vi "Project Parser.vi"(8 "error in (no error)":errorcluster, 10 "Initial Ident":i32, 11 "file path (use dialog)":path=path "C:/Users/fflores/Documents/LabVIEW Data/cRIO WFM/RT/Shared Variables/Local Variables.lvlib") -> (0 "error out":errorcluster, 2 "Item out":T1(array[cluster]))   [LabVIEW 2020, in "LV Project Items Parser.lvlib"]
doc: "This VI applies recursiveness to parse the elements of a project using its XML and return them ready to populate a tree control."
uses:
  LV Project Items Parser.lvlib
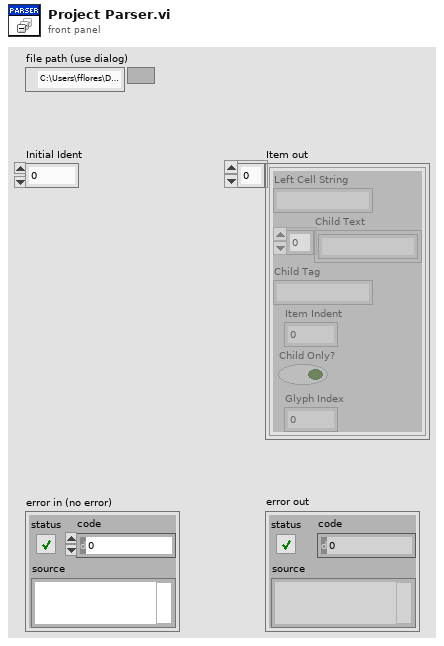
[diagram p1: front panel]
types:
  T1 = cluster{"Left Cell String":string, "Child Text":string[], "Child Tag":string, "Item Indent":i32, "Child Only?":bool, "Glyph Index":i32}[]
  T2 = cluster{"Left Cell String":string, "Child Text":string[], "Child Tag":string, "Item Indent":i32, "Child Only?":bool, "Glyph Index":i32}
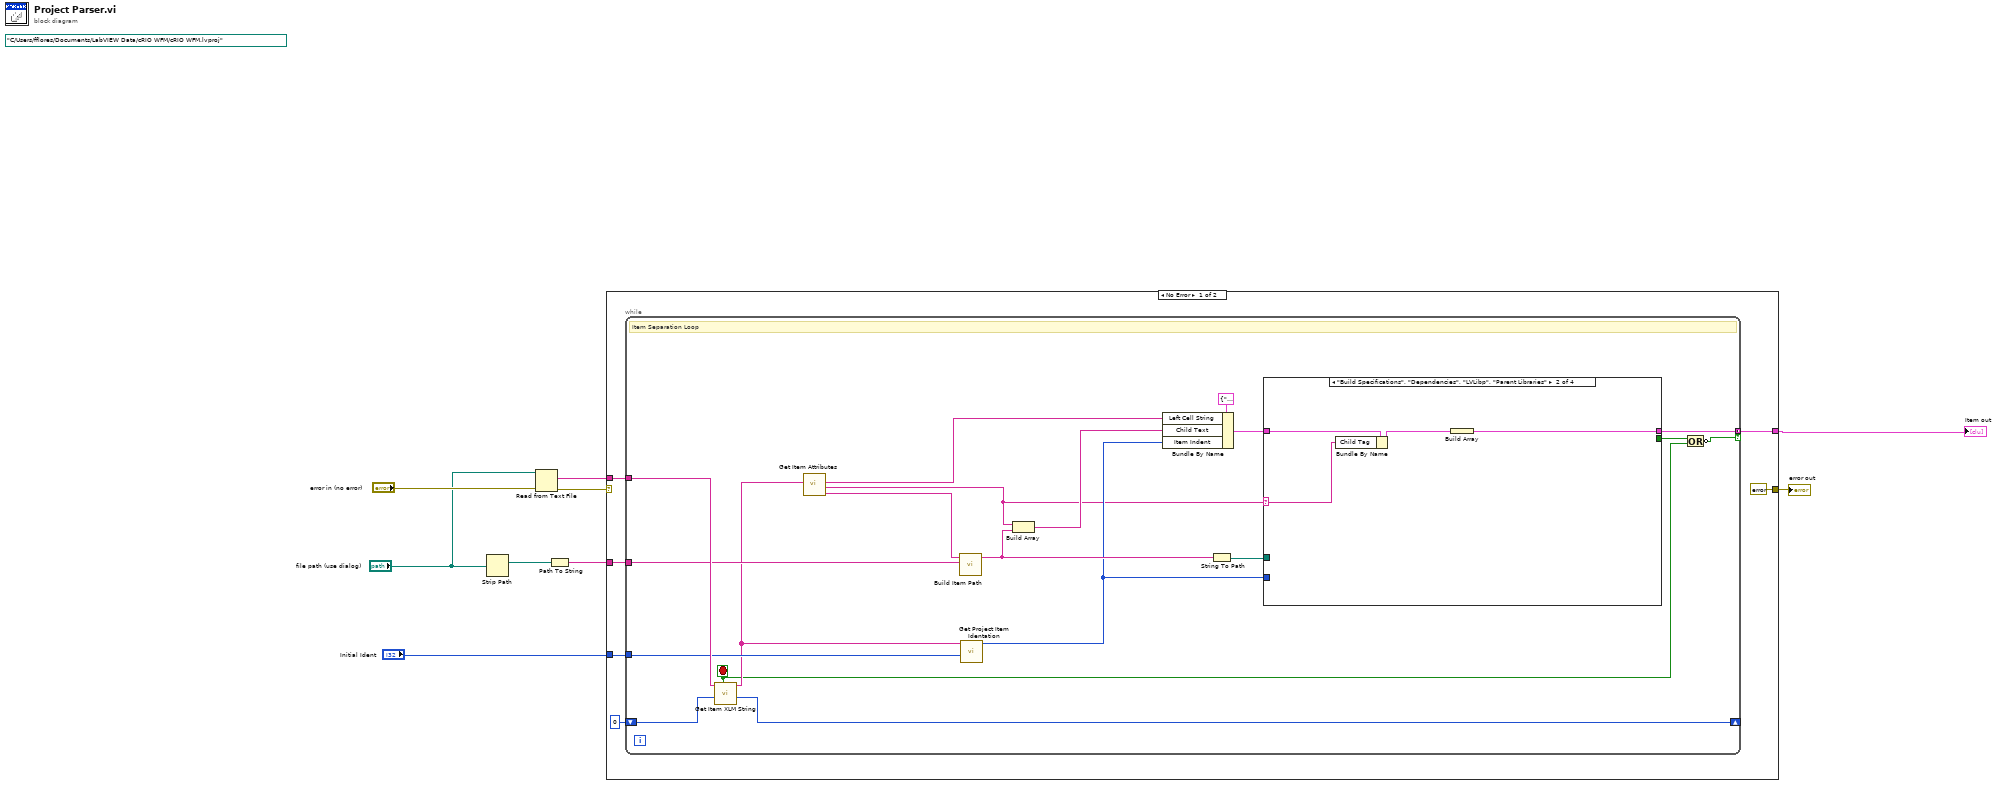
[diagram p0: block diagram]
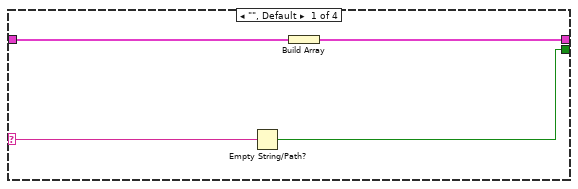
[diagram p2: hidden frame]
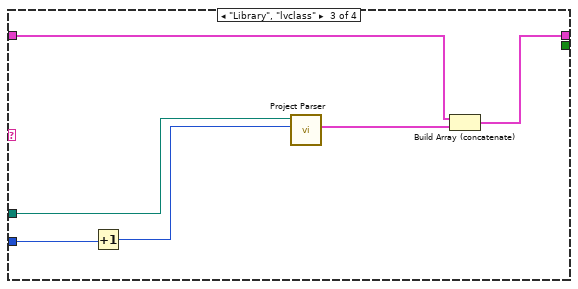
[diagram p3: hidden frame]
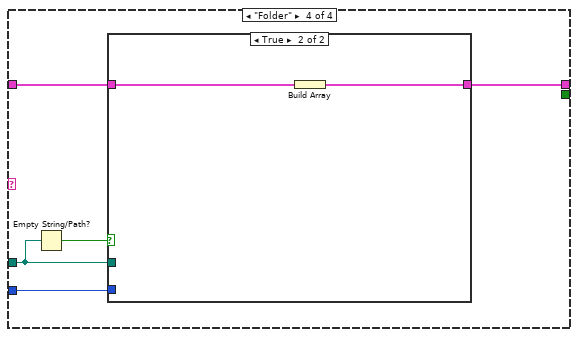
[diagram p4: hidden frame]
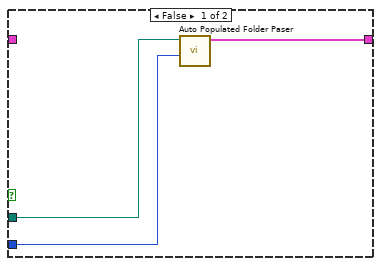
[diagram p5: hidden frame]
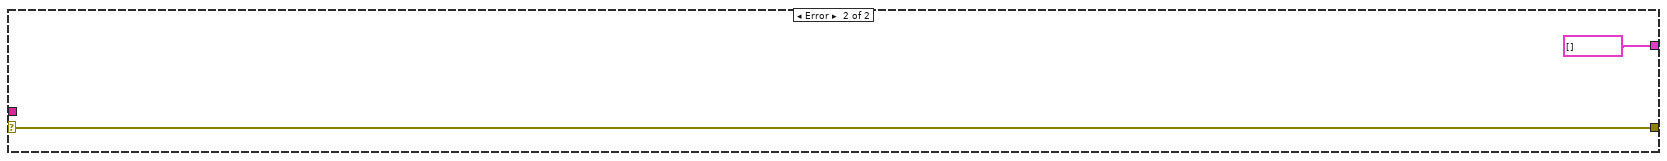
[diagram p6: hidden frame]
diagram:
  (unwired) path "C:/Users/fflores/Documents/LabVIEW Data/cRIO WFM/cRIO WFM.lvproj" ("file path (use dialog)")
  n1 = Strip Path(path="file path (use dialog)") -> (stripped path=w8:path)  [unwired: 1 out]
  n2 = Read from Text File(file (use dialog)="file path (use dialog)", error in="error in (no error)") -> (text=w7:string, error out=w2:errorcluster)  [unwired: 2 in, 2 out]
  n3 = Path To String(path=w8) -> (string=w6:string)
  n4 = case shown="No Error" w2 {
    selector: w2 -> [_ w60]
    tunnel: w7 -> [w15 _]
    tunnel: w6 -> [w14 _]
    tunnel: "Initial Ident" -> [w13 _]
    tunnel: [w11 T1 [] ("Item List Out")] -> w3
    tunnel: [errorcluster {"status"=FALSE, "code"=0, "source"=""} ("error IO") w60] -> w1
    frame No Error {
      n5 = while {
        tunnel: w15 -> [w34]
        tunnel: [w33] -> w11 mode=concatenating if=w29
        tunnel: w14 -> [w28]
        tunnel: w13 -> [w25]
        shift-right: [w23] -> _
        shift-left: 0 ("Offset Out") -> [w22]
        stop <- w17 stop-if-true
        # "Item Separation Loop"
        n6 = call "Get Item XLM String.vi"("Offset In"=w22, "XML String"=w34) -> ("Offset Out"=w23:i32, "Item XLM String"=w21:string, "Finished?"=w17:bool)  [unwired: 7 in]
        n7 = call "Get Item Attributes.vi"("Item XLM String"=w21) -> ("URL"=w20:string, "Type"=w19:string, "Item Name"=w18:string)  [unwired: 8 in]
        n8 = call "Build Item Path.vi"("Base Path"=w28, "Item URL"=w20) -> ("Item Path"=w26:string)  [unwired: 9 in]
        n9 = call "Get Project Item Identation.vi"("Initial Indent"=w25, "Item XML String"=w21) -> ("Item Ident"=w24:i32)  [unwired: 9 in]
        n10 = Build Array(w19, w26) -> (w32:string[])
        n11 = Bundle By Name(cluster=T2 {"Left Cell String"="", "Child Text"=[], "Child Tag"="", "Item Indent"=0, "Child Only?"=FALSE, "Glyph Index"=0} ("Item"), "Left Cell String"=w18, "Child Text"=w32, "Item Indent"=w24) -> (w30:T2)
        n12 = String To Path(string=w26) -> (path=w27:path)
        n13 = case shown="\"Build Specifications\", \"Dependencies\", \"LVLibp\", \"Parent Libraries\"" w19 {
          selector: w19 -> [w36 w39 _ _]
          tunnel: w24 -> [_ _ w47 w52]
          tunnel: [w37 w41 w46 w53] -> w33
          tunnel: w30 -> [w38 w42 w45 w51]
          tunnel: w27 -> [_ _ w43 w50]
          tunnel: [w35 _ _ _] -> w16
          frame "", Default {
            n14 = Empty String/Path?(string/path=w36) -> (empty?=w35:bool)
            n15 = Build Array(w38) -> (w37:T1)
          }
          frame "Build Specifications", "Dependencies", "LVLibp", "Parent Libraries" {
            n16 = Bundle By Name(cluster=w42, "Child Tag"=w39) -> (w40:T2)
            n17 = Build Array(w40) -> (w41:T1)
          }
          frame "Library", "lvclass" {
            n18 = Increment(x=w47) -> (x+1=w44:i32)
            n19 = call "Project Parser.vi"("Initial Ident"=w44, "file path (use dialog)"=w43) -> ("Item out"=w48:T1)  [unwired: 8 in, 1 out]
            n20 = Build Array (concatenate)(w45, w48) -> (w46:T1)
          }
          frame "Folder" {
            n21 = Empty String/Path?(string/path=w50) -> (empty?=w49:bool)
            n22 = case shown="True" w49 {
              tunnel: [w56 w57] -> w53
              tunnel: w52 -> [w55 _]
              tunnel: w51 -> [_ w58]
              tunnel: w50 -> [w54 _]
              frame False {
                n23 = call "Auto Populated Folder Paser.vi"("Item Indent"=w55, "path"=w54) -> ("Item List Out"=w56:T1)  [unwired: 9 in]
              }
              frame True {
                n24 = Build Array(w58) -> (w57:T1)
              }
            }
          }
        }
        n25 = Compound Arithmetic op=OR(w16, w17) -> (invert w29:bool)
      }
    }
    frame Error {
    }
  }
  "Item out" <- w3
  "error out" <- w1
